vi "Config BERT Comparator.vi"(7 "Pass Fail Limits (0.0100000)":dbl=0.01 format="%.8f", 8 "error in (no error)":errorcluster {"code" format="%.0x"}, 9 "Pass Fail Update (T:CYCLE END)":bool=TRUE, 10 "Pass Fail State (T:ON)":bool=TRUE, 11 "VISA Resource Name":refnum<visa-resource-name>) -> (0 "error out":errorcluster {"code" format="%.0x"}, 3 "VISA Resource Name Out":refnum<visa-resource-name>)   [LabVIEW 2014, in "Agilent ESG Series.lvlib"]
doc: "This VI is used to configure pass/fail judgement mode."
uses:
  Agilent ESG Series.lvlib
panel:
  # "ON"
  # "OFF"
  # "CYCLE END"
  # "FAIL HOLD"
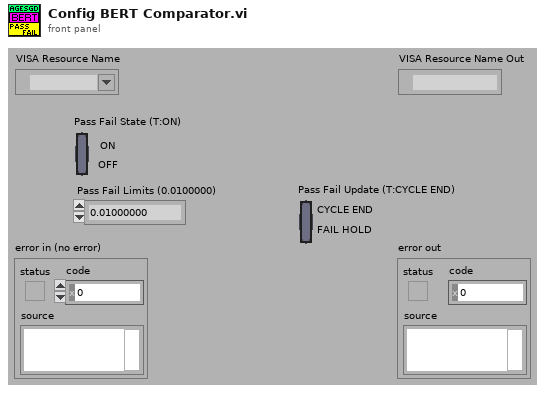
[diagram p1: front panel]
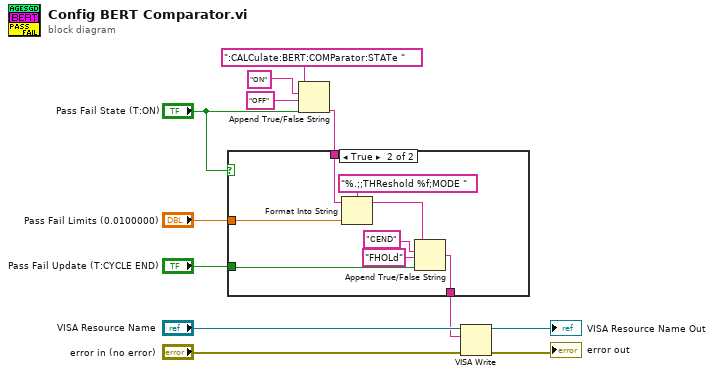
[diagram p0: block diagram]
diagram:
  n1 = Append True/False String(1:"Pass Fail State (T:ON)", 2:"OFF" ("false string"), 3:"ON" ("true string"), 4:":CALCulate:BERT:COMParator:STATe " ("string (\"\")")) -> (0:w4:string)
  n2 = case shown="True" "Pass Fail State (T:ON)" {
    tunnel: w4 -> [w13 w19]
    tunnel: "Pass Fail Limits (0.0100000)" -> [_ w18]
    tunnel: "Pass Fail Update (T:CYCLE END)" -> [_ w17]
    tunnel: [w13 w15] -> w1
    frame False {
    }
    frame True {
      n3 = Format Into String(format string="%.;;THReshold %f;MODE ", initial string=w19, w18) -> (resulting string=w16:string)  [unwired: 1 in, 1 out]
      n4 = Append True/False String(1:w17, 2:"FHOLd" ("false string"), 3:"CEND" ("true string"), 4:w16) -> (0:w15:string)
    }
  }
  n5 = VISA Write(VISA resource name="VISA Resource Name", write buffer=w1, error in (no error)="error in (no error)") -> (VISA resource name out=→"VISA Resource Name Out":refnum<visa-resource-name>, error out=→"error out":errorcluster)  [unwired: 1 out]
